vi "path steer4.vi"(11 "lane":bool) -> (2 "curve vel limit":dbl, 3 "handle":dbl=175.61695170488764)   [LabVIEW 2015]
uses:
  <vilib>/Analysis/7linalg.llb/Solve Linear Equations (single right hand).vi
  <vilib>/Analysis/baseanly.llb/Solve Linear Equations By Cholesky.vi
  <vilib>/Analysis/baseanly.llb/Real Matrix to Compact Array.vi
  <vilib>/Analysis/baseanly.llb/Real Compact Tri-Matrix Linear Eqs.vi
  G_ALL.vi
  <vilib>/Analysis/7linalg.llb/Solve Linear Eqs (General).vi
  <vilib>/Analysis/7linalg.llb/Solve Linear Eqs (Gen, single right hand).vi
  <vilib>/Analysis/NI_AALPro.lvlib
panel:
  in  "gap":dbl=3.0 format="%#_13g"
  out "cy":dbl
  out "cx":dbl
  out "slope bc":dbl
  out "slope ab":dbl
  in  "gain":dbl[](array[numeric])=[0.7, 1400.0, 750.0]
  out "R":dbl
  out "circle coeff":dbl[](array[numeric]) format="%.2f"
  out "ref":dbl[](array[numeric])
  out "circle point":dbl[][](array[numeric])
  out "map_track 2":dbl[][](array[numeric])
  in  "d lon[m] good:0.5":dbl format="%#_13g"
  out "appended array":dbl[](array[numeric])
  out "range":dbl[](graph)
  out "path end":bool
  in  "an[g]":dbl=-0.17 format="%#_13g"
  out "Waveform Graph":dynamicdata(graph)
  in  "mu":dbl=0.005 format="%#_13g"
  out "x":dbl=-0.8542483758567541
  out "XY Graph":cluster{"Y":dbl[], "Y":dbl[]}[](graph)=[{"Y"=[-5.246809304707959, -4.763210909809536, -4.298248751776158, -3.853163667485589, -3.4268765479315446, -3.029477672753705, -2.6673284986480974, -2.335336691519628, -2.0366453167866156, -1.7750835921098853, -1.5528767688369498, -1.3644656447475765, -1.2079630605299954, -1.074690008661569, -0.9585132340675446, -0.8551782329420596, -0.7665829934540727, -0.6868993462607671, -0.6126823280970868, -0.5442164343365972, -0.47614894814750475, -0.41410047141640827, -0.3538150238541624, -0.29540366128691464, -0.24219086500490516, -0.19691528446819184, -0.15547027846011519, -0.11340295527325328, -0.07144915398020535, -0.03434793001665748, 0.0, 0.026526158792223087, 0.05124494389382517, 0.07270742281515652, 0.06435385726912624, -0.004553363938687882, -0.139882839282637, -0.3359547912247316, -0.5900103181212502, -0.900040761768828, -1.2577413584671457, -1.66216965308078, -2.1012210225275174, -2.5653232377446606, -3.0450206197370466, -3.5404770109177743, -4.039369871326692, -4.541851143281866, -5.046387603513992, -5.553897537492966, -6.061637927692216, -6.567645563226444, -7.068648217182836, -7.570715384980373, -8.064438697718192, -8.545111556606587, -8.998477174205098, -9.422019565773061, -9.805695724849244, -10.146105279341642], "Y"=[-13.12635530502614, -12.964543503689939, -12.76763447744193, -12.524937360608902, -12.2475735581719, -11.933583222485607, -11.583671941038977, -11.206464906204559, -10.79245190322264, -10.354599285401152, -9.898639757724679, -9.426030687571156, -8.945680321385996, -8.454465203163156, -7.963985068856038, -7.468786738899853, -6.97312085053041, -6.479311060157665, -5.971731167568438, -5.469535412616666, -4.9636888467403155, -4.464752828537232, -3.9649913085777393, -3.458342585235778, -2.9601418499725303, -2.459972000641257, -1.9586644185731306, -1.4494467342092758, -0.9454480119816643, -0.4403687170997531, 0.06136222931732077, 0.5678735764406926, 1.068808881478275, 1.5686590067794068, 2.0720530905057277, 2.5736288544042853, 3.0594879994083963, 3.5248827445502124, 3.9579216058298154, 4.3560080630331335, 4.707794061133773, 5.011781058067703, 5.259264085768475, 5.451142759582283, 5.593309208559008, 5.693936293621469, 5.758617125078806, 5.791664966026638, 5.794000380643315, 5.784136801290129, 5.782533687658117, 5.785062966223215, 5.79993550563809, 5.8290421589798, 5.9156579447766475, 6.067163605595132, 6.278887512503447, 6.54911596168099, 6.871713294872911, 7.24413426029683]}, {"Y"=[-27.79054311036769, -27.788426793206575, -27.782078486373944, -27.77150012362555, -27.75669492723317, -27.737667407003034, -27.71442335890214, -27.686969863292695, -27.655315282775426, -27.619469259642194, -27.5794427129389, -27.5352478351394, -27.48689808843162, -27.434408200616765, -27.377794160623147, -27.317073213635787, -27.25226385584335, -27.18338582880404, -27.110460113432133, -27.033508923606977, -26.95255569940644, -26.867625099966816, -26.77874299597144, -26.68593646177021, -26.589233767132484, -26.488664368635824, -26.384258900693254, -26.2760491662217, -26.16406812695454, -26.048349893401117, -25.92892971445636, -25.805843966663623, -25.679130143134046, -25.548826842125777, -25.41497375528658, -25.27761165556337, -25.13678238478238, -24.992528840903734, -24.844894964954314, -24.693925727642892, -24.53966711566163, -24.382166117678068, -24.221470710021944, -24.057629842071115, -23.890693421341133, -23.720712298282884, -23.547738250793113, -23.37182396844231, -23.193023036425007, -23.011389919237175, -22.82697994408583, -22.639849284035826, -22.450054940898987, -22.257654727870808, -22.062707251920006, -21.865271895936253, -21.66540880064158, -21.463178846270928, -21.25864363402745, -21.05186546731817, -20.84290733277577, -20.631832881072256, -20.41870640753034, -20.20359283253847, -19.986557681775434, -19.767667066250628, -19.54698766216598, -19.324586690605734, -19.10053189706029, -18.874891530790215, -18.64773432403691, -18.419129471086073, -18.18914660719046, -17.957855787358298, -17.725327465013883, -17.491632470536747, -17.256841989686063, -17.02102754191677, -16.784260958594032, -16.546614361112756, -16.308160138928653, -16.068970927507767, -15.829119586200973, -15.588679176050324, -15.347722937533948, -15.106324268256303, -14.864556700590517, -14.622493879279771, -14.38020953900434, -14.137777481921338, -13.895271555183845, -13.652765628446353, -13.410333571363354, -13.16804923108792, -12.92598640977717, -12.684218842111388, -12.442820172833741, -12.20186393431737, -11.961423524166722, -11.721572182859921, -11.482382971439037, -11.243928749254936, -11.006282151773657, -10.769515568450924, -10.533701120681629, -10.298910639830943, -10.06521564535381, -9.832687323009392, -9.601396503177233, -9.37141363928162, -9.142808786330779, -8.915651579577474, -8.690011213307402, -8.465956419761957, -8.243555448201716, -8.022876044117066, -7.803985428592254, -7.586950277829223, -7.371836702837354, -7.158710229295436, -6.947635777591925, -6.738677643049522, -6.531899476340242, -6.32736426409676, -6.125134309726112, -5.925271214431441, -5.727835858447683, -5.53288838249688, -5.3404881694687045, -5.150693826331867, -4.96356316628186, -4.779153191130517, -4.597520073942688, -4.418719141925381, -4.242804859574576, -4.069830812084804, -3.8998496890265617, -3.7329132682965724, -3.5690724003457444, -3.4083769926896217, -3.250875994706062, -3.096617382724796, -2.9456481454133776, -2.798014269463957, -2.6537607255853093, -2.5129314548043187, -2.3755693550811117, -2.241716268241916, -2.1114129672336457, -1.9846991437040682, -1.8616133959113306, -1.7421932169665748, -1.62647498341315, -1.5144939441459915, -1.406284209674439, -1.3018787417318656, -1.201309343235204, -1.1046066485974766, -1.0118001143962498, -0.9229180104008776, -0.8379874109612526, -0.7570341867607127, -0.6800829969355568, -0.6071572815636515, -0.5382792545243404, -0.47346989673190265, -0.41274894974454135, -0.3561349097509261, -0.30364502193607024, -0.25529527522828666, -0.21110039742879394, -0.1710738507254952, -0.13522782759226182, -0.10357324707499238, -0.07611975146555316, -0.052875703364655635, -0.03384818313452165, -0.019042986742137558, -0.00846462399374559, -0.0021163171611142673, 0.0, -0.0021163171611142673, -0.00846462399374559, -0.019042986742137558, -0.03384818313452165, -0.052875703364655635, -0.07611975146555316, -0.10357324707499238, -0.13522782759226182, -0.17107385072549341, -0.21110039742879394, -0.25529527522828666, -0.30364502193607024, -0.3561349097509261, -0.4127489497445396, -0.4734698967319009, -0.5382792545243387, -0.6071572815636497, -0.6800829969355586, -0.7570341867607127, -0.8379874109612526, -0.9229180104008758, -1.011800114396248, -1.1046066485974766, -1.2013093432352022, -1.3018787417318638, -1.4062842096744355, -1.5144939441459861, -1.6264749834131482, -1.7421932169665766, -1.8616133959113323, -1.9846991437040664, -2.111412967233644, -2.2417162682419143, -2.37556935508111, -2.512931454804317, -2.6537607255853075, -2.798014269463952, -2.9456481454133705, -3.0966173827247943, -3.2508759947060604, -3.4083769926896235, -3.569072400345746, -3.7329132682965707, -3.89984968902656, -4.069830812084803, -4.242804859574575, -4.418719141925379, -4.597520073942681, -4.77915319113051, -4.9635631662818565, -5.150693826331869, -5.340488169468708, -5.532888382496882, -5.727835858447682, -5.925271214431433, -6.125134309726104, -6.3273642640967624, -6.531899476340239, -6.738677643049519, -6.947635777591917, -7.158710229295428, -7.371836702837351, -7.58695027782922, -7.803985428592251, -8.022876044117067, -8.243555448201715, -8.465956419761955, -8.6900112133074, -8.915651579577467, -9.14280878633077, -9.371413639281617, -9.601396503177229, -9.832687323009386, -10.065215645353812, -10.298910639830945, -10.533701120681625, -10.769515568450919, -11.006282151773648, -11.24392874925494, -11.482382971439037, -11.721572182859921, -11.961423524166714, -12.201863934317359, -12.442820172833729, -12.684218842111388, -12.925986409777169, -13.168049231087927, -13.410333571363354, -13.652765628446351, -13.895271555183843, -14.137777481921333, -14.380209539004332, -14.622493879279759, -14.864556700590516, -15.106324268256296, -15.347722937533955, -15.588679176050325, -15.82911958620097, -16.068970927507763, -16.30816013892865, -16.546614361112745, -16.784260958594036, -17.021027541916766, -17.25684198968606, -17.49163247053674, -17.725327465013873, -17.957855787358298, -18.189146607190455, -18.41912947108607, -18.647734324036914, -18.874891530790215, -19.100531897060286, -19.32458669060573, -19.546987662165968, -19.767667066250617, -19.986557681775434, -20.203592832538465, -20.418706407530333, -20.631832881072256, -20.842907332775766, -21.051865467318166, -21.258643634027447, -21.46317884627092, -21.66540880064158, -21.865271895936253, -22.062707251920003, -22.257654727870804, -22.45005494089898, -22.63984928403582, -22.826979944085828, -23.01138991923717, -23.19302303642501, -23.371823968442314, -23.54773825079311, -23.720712298282884, -23.890693421341126, -24.057629842071112, -24.221470710021936, -24.382166117678068, -24.539667115661626, -24.693925727642895, -24.844894964954314, -24.992528840903734, -25.13678238478238, -25.277611655563366, -25.414973755286574, -25.548826842125777, -25.679130143134046, -25.805843966663623, -25.928929714456356, -26.04834989340111, -26.16406812695454, -26.276049166221696, -26.384258900693247, -26.488664368635824, -26.589233767132484, -26.68593646177021, -26.778742995971438, -26.867625099966812, -26.95255569940643, -27.033508923606977, -27.110460113432133, -27.183385828804038, -27.25226385584335, -27.317073213635787, -27.377794160623147, -27.434408200616765, -27.486898088431616, -27.535247835139405, -27.5794427129389, -27.619469259642194, -27.655315282775426, -27.686969863292695, -27.71442335890214, -27.737667407003034, -27.75669492723317, -27.77150012362555, -27.782078486373944, -27.788426793206575], "Y"=[-0.0, -0.24250592673749302, -0.48493798382049413, -0.7272223240959237, -0.969285145406673, -1.2110527130724553, -1.4524513823501046, -1.6934076208664777, -1.9338480310171269, -2.1736993723239215, -2.4128885837448077, -2.6513428059289086, -2.8889894034101893, -3.1257559867329223, -3.3615704345022186, -3.596360915352901, -3.830055909830037, -4.062584232174453, -4.293875052006613, -4.52385791590223, -4.752462768853066, -4.97961997560637, -5.205260341876442, -5.429315135421889, -5.65171610698213, -5.872395511066782, -6.091286126591589, -6.308321277354623, -6.523434852346495, -6.736561325888409, -6.9476357775919215, -7.156593912134322, -7.363372078843605, -7.567907291087082, -7.770137245457733, -7.970000340752407, -8.167435696736161, -8.362383172686963, -8.55478338571514, -8.744577728851981, -8.931708388901985, -9.11611836405333, -9.29775148124116, -9.476552413258466, -9.652466695609267, -9.82544074309904, -9.995421866157285, -10.162358286887272, -10.326199154838099, -10.486894562494223, -10.644395560477784, -10.798654172459047, -10.949623409770469, -11.09725728571989, -11.241510829598536, -11.382340100379524, -11.519702200102733, -11.65355528694193, -11.783858587950201, -11.910572411479777, -12.033658159272512, -12.15307833821727, -12.268796571770693, -12.380777611037853, -12.488987345509406, -12.59339281345198, -12.693962211948639, -12.790664906586368, -12.883471440787595, -12.97235354478297, -13.057284144222592, -13.138237368423132, -13.215188558248288, -13.288114273620195, -13.356992300659504, -13.421801658451942, -13.482522605439303, -13.539136645432919, -13.591626533247775, -13.639976279955558, -13.684171157755053, -13.72419770445835, -13.760043727591583, -13.791698308108852, -13.819151803718292, -13.84239585181919, -13.861423372049323, -13.876228568441707, -13.8868069311901, -13.89315523802273, -13.895271555183845, -13.89315523802273, -13.8868069311901, -13.876228568441707, -13.861423372049323, -13.84239585181919, -13.819151803718293, -13.791698308108852, -13.760043727591583, -13.72419770445835, -13.684171157755053, -13.639976279955558, -13.591626533247775, -13.53913664543292, -13.482522605439303, -13.421801658451942, -13.356992300659504, -13.288114273620195, -13.215188558248288, -13.138237368423134, -13.057284144222592, -12.972353544782969, -12.883471440787595, -12.790664906586368, -12.69396221194864, -12.593392813451981, -12.488987345509406, -12.380777611037855, -12.268796571770697, -12.153078338217272, -12.033658159272516, -11.910572411479778, -11.783858587950201, -11.65355528694193, -11.519702200102735, -11.382340100379528, -11.241510829598536, -11.09725728571989, -10.949623409770469, -10.79865417245905, -10.644395560477784, -10.486894562494225, -10.326199154838102, -10.162358286887274, -9.995421866157285, -9.825440743099042, -9.65246669560927, -9.476552413258466, -9.297751481241159, -9.11611836405333, -8.931708388901988, -8.74457772885198, -8.554783385715142, -8.362383172686968, -8.167435696736163, -7.9700003407524065, -7.770137245457734, -7.567907291087087, -7.363372078843605, -7.1565939121343245, -6.9476357775919215, -6.7365613258884105, -6.523434852346494, -6.308321277354625, -6.091286126591593, -5.872395511066783, -5.6517161069821285, -5.42931513542189, -5.205260341876445, -4.979619975606376, -4.752462768853069, -4.523857915902228, -4.293875052006615, -4.062584232174458, -3.8300559098300377, -3.596360915352905, -3.361570434502219, -3.1257559867329254, -2.888989403410189, -2.6513428059289113, -2.4128885837448126, -2.1736993723239233, -1.933848031017125, -1.6934076208664786, -1.4524513823501084, -1.2110527130724555, -0.969285145406676, -0.7272223240959296, -0.4849379838204965, -0.24250592673749197, -1.7016237834565482e-15, 0.24250592673748858, 0.4849379838204931, 0.72722232409592, 0.9692851454066664, 1.2110527130724522, 1.4524513823501048, 1.6934076208664814, 1.9338480310171278, 2.1736993723239197, 2.4128885837448095, 2.6513428059289077, 2.8889894034101857, 3.1257559867329223, 3.3615704345022155, 3.5963609153528955, 3.830055909830029, 4.062584232174455, 4.293875052006618, 4.523857915902231, 4.752462768853065, 4.979619975606372, 5.205260341876442, 5.429315135421887, 5.651716106982125, 5.872395511066779, 6.0912861265915845, 6.308321277354616, 6.52343485234649, 6.736561325888413, 6.947635777591924, 7.156593912134322, 7.363372078843602, 7.567907291087084, 7.7701372454577315, 7.970000340752404, 8.16743569673616, 8.36238317268696, 8.554783385715135, 8.744577728851977, 8.931708388901985, 9.116118364053332, 9.29775148124116, 9.476552413258464, 9.652466695609267, 9.825440743099039, 9.995421866157281, 10.162358286887272, 10.326199154838095, 10.48689456249422, 10.644395560477783, 10.798654172459052, 10.94962340977047, 11.09725728571989, 11.241510829598534, 11.382340100379523, 11.51970220010273, 11.653555286941932, 11.7838585879502, 11.910572411479777, 12.03365815927251, 12.153078338217266, 12.268796571770695, 12.380777611037853, 12.488987345509404, 12.593392813451981, 12.69396221194864, 12.790664906586366, 12.883471440787595, 12.972353544782967, 13.057284144222589, 13.138237368423132, 13.215188558248288, 13.288114273620193, 13.356992300659506, 13.421801658451942, 13.482522605439303, 13.539136645432919, 13.591626533247773, 13.63997627995556, 13.684171157755053, 13.72419770445835, 13.760043727591581, 13.791698308108852, 13.819151803718292, 13.84239585181919, 13.861423372049323, 13.876228568441707, 13.8868069311901, 13.89315523802273, 13.895271555183845, 13.89315523802273, 13.8868069311901, 13.876228568441707, 13.861423372049323, 13.84239585181919, 13.819151803718292, 13.791698308108852, 13.760043727591583, 13.724197704458351, 13.684171157755053, 13.63997627995556, 13.591626533247773, 13.539136645432919, 13.482522605439305, 13.421801658451944, 13.356992300659506, 13.288114273620195, 13.21518855824829, 13.138237368423134, 13.05728414422259, 12.972353544782969, 12.883471440787597, 12.79066490658637, 12.693962211948643, 12.593392813451985, 12.488987345509408, 12.380777611037855, 12.268796571770697, 12.15307833821727, 12.033658159272512, 11.910572411479778, 11.783858587950203, 11.653555286941934, 11.519702200102733, 11.382340100379524, 11.241510829598537, 11.097257285719893, 10.949623409770474, 10.798654172459056, 10.644395560477784, 10.486894562494227, 10.326199154838095, 10.16235828688727, 9.995421866157285, 9.825440743099042, 9.65246669560927, 9.47655241325847, 9.29775148124117, 9.11611836405333, 8.931708388901988, 8.744577728851976, 8.554783385715139, 8.362383172686963, 8.167435696736165, 7.970000340752413, 7.770137245457741, 7.567907291087083, 7.363372078843606, 7.156593912134326, 6.947635777591929, 6.736561325888418, 6.523434852346495, 6.308321277354626, 6.091286126591594, 5.872395511066778, 5.65171610698213, 5.429315135421891, 5.205260341876446, 4.979619975606377, 4.752462768853076, 4.52385791590223, 4.293875052006616, 4.062584232174459, 3.8300559098300337, 3.5963609153529004, 3.3615704345022204, 3.125755986732927, 2.888989403410197, 2.651342805928907, 2.4128885837448086, 2.173699372323925, 1.9338480310171329, 1.6934076208664863, 1.4524513823501162, 1.2110527130724573, 0.9692851454066778, 0.7272223240959189, 0.484937983820492, 0.24250592673749366]}]
  # "d lon : 경로 위 3점 위치 밀기"
  # "mu : 마찰력\nan :  감가속도"
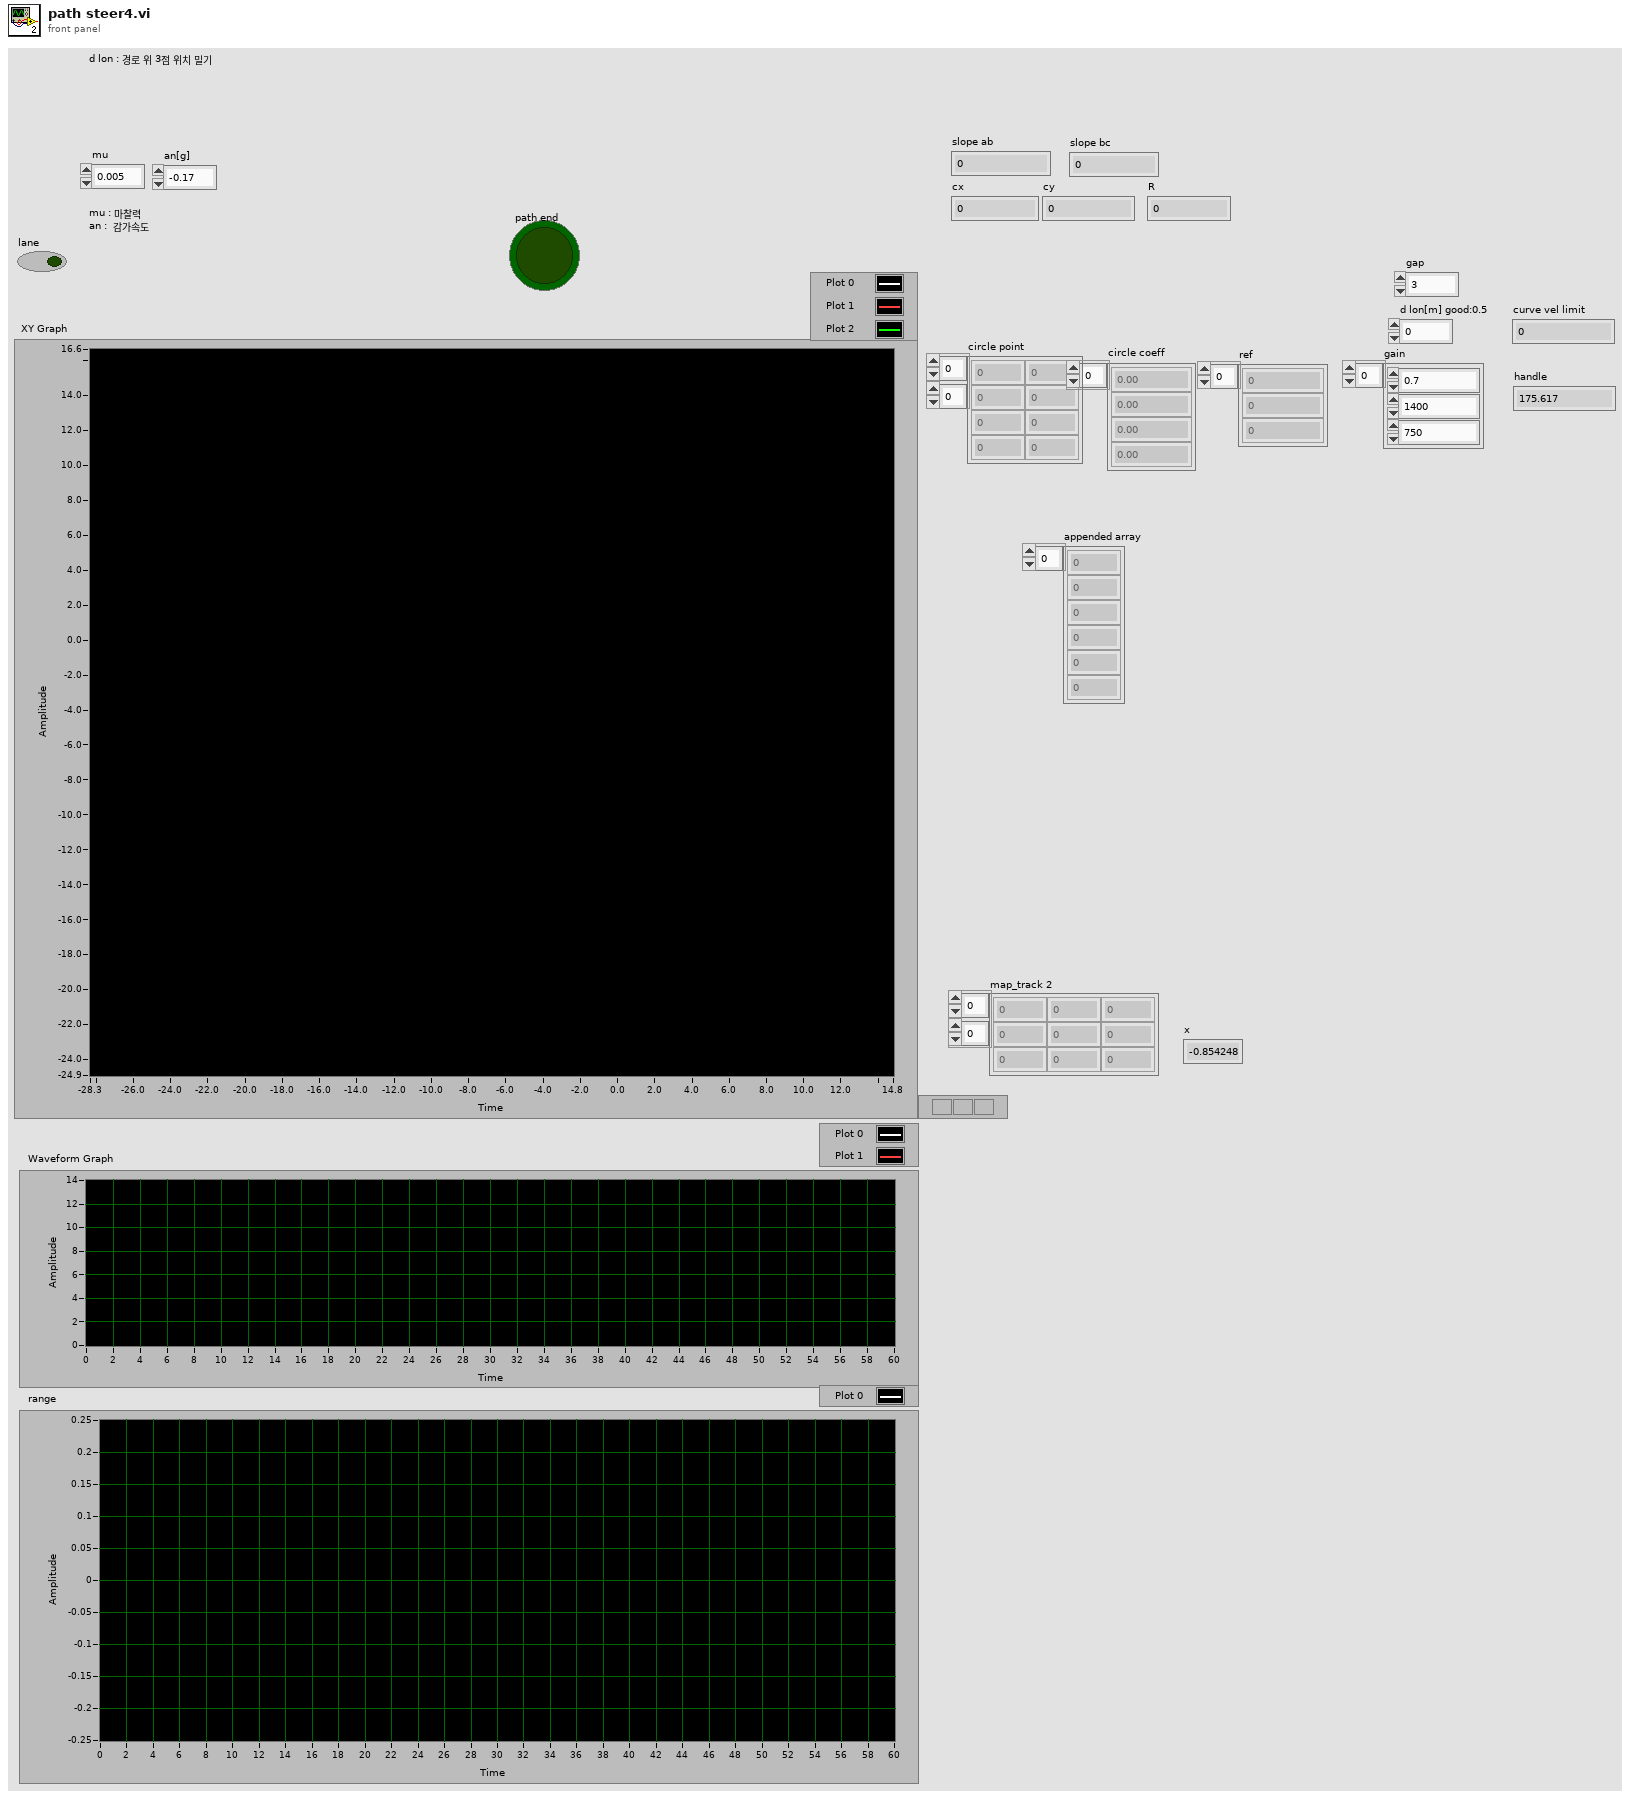
[diagram p1: front panel]
types:
  T1 = cluster{"Steer_input":dbl, "Steer_output":dbl, "VS_des":dbl, "VS_can":dbl, "heading":dbl, "auto":bool, "run":bool, "x":dbl, "y":dbl, "slam_y":dbl, "slam_x":dbl, "slam_heading":dbl}
  T2 = cluster{"C_Wheel base":dbl, "ratio_steer":dbl, "Overall width":dbl, "af":dbl, "turn radius":dbl, "eval":dbl, "ap":dbl, "an":dbl, "Vmax":dbl, "mu":dbl, "Vlast":dbl}
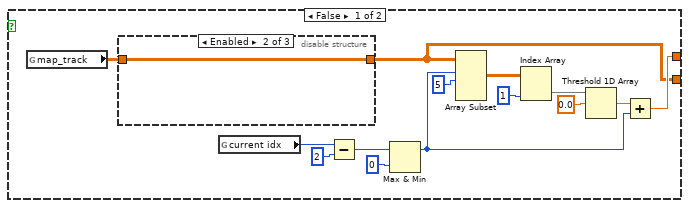
[diagram p2: hidden frame]
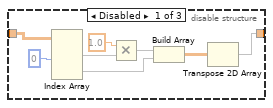
[diagram p3: hidden frame]
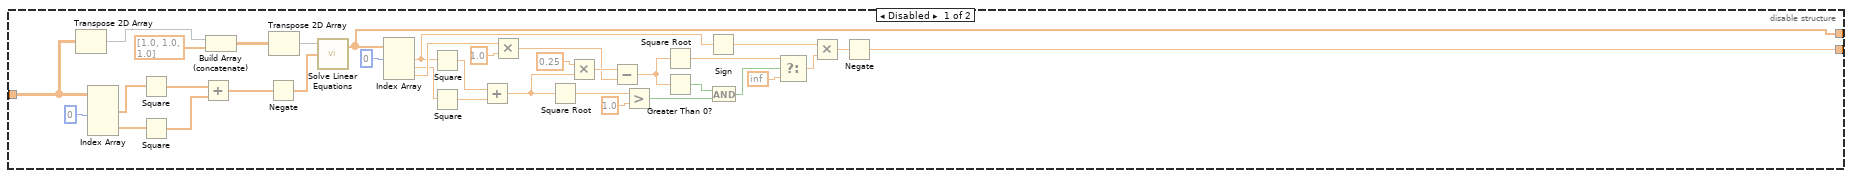
[diagram p6: hidden frame]
diagram:
  n1 = flat-sequence {
    tunnel: [w10] -> w9
    tunnel: w9 -> [w111]
    tunnel: [w124] -> w8
    tunnel: [w118] -> w7
    tunnel: [w111] -> w6
    tunnel: w8 -> [w279]
    tunnel: [w279] -> w5
    tunnel: w7 -> [w278]
    tunnel: [w278] -> w3
    tunnel: w6 -> [w264]
    tunnel: w5 -> [w458]
    tunnel: [w458] -> w4
    tunnel: w3 -> [w457]
    tunnel: [w457] -> w2
    tunnel: [w418] -> w1
    tunnel: w4 -> [w461]
    tunnel: w2 -> [w460]
    tunnel: w1 -> [w459]
    frame #0 {
      n2 = case shown="True" "lane" {
        tunnel: [w66 w89] -> w56
        tunnel: [w68 _] -> w19
        frame False {
          n3 = global read "G_ALL.vi" "map_track"() -> (w67:dbl[][])
          n4 = disable-structure shown="Enabled" {
            disable-tunnel: w67 -> [w87 w88 _]
            disable-tunnel: [w80 w88 _] -> w66
            frame Disabled {
              n5 = Index Array(array=w87, index (col) #1=0 ("disabled index (col)")) -> (element #1=w85:dbl[], element #2=w82:dbl[])  [unwired: 3 in]
              n6 = Multiply(x=1.0, y=w85) -> (x*y=w83:dbl[])
              n7 = Build Array(w83, w82) -> (w81:dbl[][])
              n8 = Transpose 2D Array(2D array=w81) -> (transposed array=w80:dbl[][])
            }
            frame Enabled {
            }
            frame Disabled {
            }
          }
          n9 = global read "G_ALL.vi" "current idx"() -> (w69:i32)
          n10 = Subtract(x=w69, y=2) -> (x-y=w78:i32)
          n11 = Max & Min(x=w78, y=0) -> (max(x,y)=w72:i32)  [unwired: 1 out]
          n12 = Array Subset(array=w66, index (row)=w72, length (row)=5 ("length")) -> (w75:dbl[][])  [unwired: 2 in]
          n13 = Index Array(array=w75, index (col)=1 ("disabled index (col)")) -> (element=w73:dbl[])  [unwired: 1 in]
          n14 = Threshold 1D Array(2:0.0 ("threshold y"), 3:w73) -> (0:w70:dbl)  [unwired: 1 in]
          n15 = Add(x=w70, y=w72) -> (x+y=w68:dbl)
        }
        frame True {
          n16 = global read "G_ALL.vi" "map_track lane"() -> (w89:dbl[][])
        }
      }
      n17 = Round Toward +Infinity(x=w19) -> (ceil(x): smallest int >= x=w27:dbl)
      n18 = Round Toward -Infinity(1:w19) -> (0:w26:dbl)
      n19 = Index Array(array=w56, index (col) #1=0 ("disabled index (col)")) -> (element #1=w64:dbl[], element #2=w63:dbl[])  [unwired: 3 in]
      n20 = Equal?(x=w26, y=w19) -> (x = y?=w25:bool)
      n21 = To Long Integer(number=w26) -> (32bit integer=w23:i32)
      n22 = Interpolate 1D Array(1:w19, 2:w64) -> (0:w62:dbl)
      n23 = Interpolate 1D Array(1:w19, 2:w63) -> (0:w61:dbl)
      n24 = Increment(x=w23) -> (x+1=w22:i32)
      n25 = To Long Integer(number=w27) -> (32bit integer=w21:i32)
      n26 = Select(t=w23, s=w25, f=w22) -> (s? t:f=w24:i32)
      n27 = global read "G_ALL.vi" "CARDATA"() -> (w58:T1)
      n28 = Array Subset(array=w56, index (row)=0 ("index"), length (row)=w24) -> (w54:dbl[][])  [unwired: 2 in]
      n29 = Unbundle By Name(w58) -> ("VS_can"=w18:dbl)
      n30 = Index Array(array=w54, index (col) #1=0 ("disabled index (col)")) -> (element #1=w52:dbl[], element #2=w51:dbl[])  [unwired: 3 in]
      n31 = Reverse 1D Array(array=w52) -> (reversed array=w50:dbl[])
      n32 = Reverse 1D Array(array=w51) -> (reversed array=w49:dbl[])
      n33 = Multiply(x=2.0, y=w18) -> (x*y=w17:dbl)
      n34 = Build Array(w50, w49) -> (w29:dbl[][])
      n35 = Max & Min(x=w17, y=25.0) -> (max(x,y)=w57:dbl)  [unwired: 1 out]
      n36 = Transpose 2D Array(2D array=w29) -> (transposed array=w28:dbl[][])
      n37 = Build Array(w62, w61) -> (w47:dbl[])
      n38 = Array Subset(array=w56, index (row)=w21) -> (w31:dbl[][])  [unwired: 3 in]
      n39 = for {
        tunnel: w28 -> [w92] mode=indexing
        shift-right: [w92] -> _
        shift-left: w47 -> [w99]
        shift-right: [w91] -> _
        shift-left: 0.0 -> [w94]
        tunnel: 15.0 ("y") -> [w93]
        tunnel: [w91] -> w43 mode=indexing
        stop <- w90 stop-if-true
        n40 = Subtract(x=w92, y=w99) -> (x-y=w98:dbl[])
        n41 = Square(x=w98) -> (x^2=w97:dbl[])
        n42 = Add Array Elements(numeric array=w97) -> (sum=w96:dbl)
        n43 = Square Root(x=w96) -> (sqrt(x)=w95:dbl)
        n44 = Add(x=w94, y=w95) -> (x+y=w91:dbl)
        n45 = Greater Or Equal?(x=w91, y=w93) -> (x >= y?=w90:bool)
      }
      n46 = for {
        tunnel: w31 -> [w102] mode=indexing
        shift-right: [w102] -> _
        shift-left: w47 -> [w109]
        shift-right: [w101] -> _
        shift-left: 0.0 -> [w104]
        tunnel: w57 -> [w103]
        tunnel: [w101] -> w30 mode=indexing
        tunnel: [w100] -> w13
        stop <- w100 stop-if-true
        n47 = Subtract(x=w102, y=w109) -> (x-y=w108:dbl[])
        n48 = Square(x=w108) -> (x^2=w107:dbl[])
        n49 = Add Array Elements(numeric array=w107) -> (sum=w106:dbl)
        n50 = Square Root(x=w106) -> (sqrt(x)=w105:dbl)
        n51 = Add(x=w104, y=w105) -> (x+y=w101:dbl)
        n52 = Greater Or Equal?(x=w101, y=w103) -> (x >= y?=w100:bool)
      }
      n53 = Not(x=w13) -> (.not. x?=→"path end":bool)
      n54 = Negate(x=w43) -> (-x=w45:dbl[])
      n55 = Array Size(array=w43) -> (size(s)=w41:i32)
      n56 = Array Size(array=w30) -> (size(s)=w14:i32)
      n57 = Reverse 1D Array(array=w45) -> (reversed array=w44:dbl[])
      n58 = Array Subset(array=w28, index (row)=0 ("index"), length (row)=w41) -> (w36:dbl[][])  [unwired: 2 in]
      n59 = Array Subset(array=w31, index (row)=0 ("index"), length (row)=w14) -> (w15:dbl[][])  [unwired: 2 in]
      n60 = Build Array (concatenate)(w44, w30) -> (w10:dbl[])
      n61 = Index Array(array=w36, index (col) #1=0 ("disabled index (col)")) -> (element #1=w35:dbl[], element #2=w34:dbl[])  [unwired: 3 in]
      n62 = Reverse 1D Array(array=w35) -> (reversed array=w38:dbl[])
      n63 = Reverse 1D Array(array=w34) -> (reversed array=w39:dbl[])
      n64 = Build Array(w38, w39) -> (w40:dbl[][])
      n65 = Transpose 2D Array(2D array=w40) -> (transposed array=w33:dbl[][])
      n66 = Build Array (concatenate)(w33, w15) -> (w11:dbl[][])
      "map_track 2" <- w11
      n67 = global write "G_ALL.vi" "dist"(w10) -> ()
      n68 = global write "G_ALL.vi" "map_track 2"(w11) -> ()
    }
    frame #1 {
      n69 = Threshold 1D Array(2:0.0 ("threshold y"), 3:w111) -> (0:w152:dbl)  [unwired: 1 in]
      n70 = local read "map_track 2"() -> (w110:dbl[][])
      n71 = Index Array(array=w110, index (col) #1=0 ("disabled index (col)"), index (col) #3=0 ("index (col)")) -> (element #1=w159:dbl[], element #2=w151:dbl[], element #3=w149:dbl[])  [unwired: 4 in]
      n72 = Array Size(array=w151) -> (size(s)=w158:i32)
      n73 = Interpolate 1D Array(1:w152, 2:w149) -> (0:→"x":dbl)
      n74 = Decrement(x=w158) -> (x-1=w157:i32)
      n75 = for {
        tunnel: w111 -> [w194]
        tunnel: w111 -> [w239] mode=indexing
        tunnel: w159 -> [w191]
        tunnel: w151 -> [w190]
        tunnel: [w207] -> w156 mode=indexing
        tunnel: w157 -> [w206]
        tunnel: [w184] -> w155 mode=indexing
        tunnel: [w187] -> w115
        tunnel: 5.0 ("x") -> [w192]
        tunnel: [w186] -> _ mode=indexing
        i -> [w187]
        stop <- w205 stop-if-true
        n76 = Add(x=w239, y=w192) -> (x+y=w186:dbl)
        n77 = Add(x=w186, y=w192) -> (x+y=w193:dbl)
        n78 = Index Array(array=w191, index=w187) -> (element=w233:dbl)
        n79 = Index Array(array=w190, index=w187) -> (element=w232:dbl)
        n80 = Threshold 1D Array(1:w187, 2:w186, 3:w194) -> (0:w238:dbl)
        n81 = Threshold 1D Array(1:w187, 2:w193, 3:w194) -> (0:w188:dbl)
        n82 = Interpolate 1D Array(1:w238, 2:w191) -> (0:w185:dbl)
        n83 = Interpolate 1D Array(1:w238, 2:w190) -> (0:w237:dbl)
        n84 = Greater Or Equal?(x=w188, y=w206) -> (x >= y?=w205:bool)
        n85 = Interpolate 1D Array(1:w188, 2:w191) -> (0:w236:dbl)
        n86 = Interpolate 1D Array(1:w188, 2:w190) -> (0:w235:dbl)
        n87 = Build Array(w233, w232) -> (w201:dbl[])
        n88 = Build Array(w236, w235) -> (w234:dbl[])
        n89 = Build Array(w185, w237) -> (w189:dbl[])
        n90 = Build Array(w201, w189, w234) -> (w204:dbl[][])
        n91 = Build Array(w189, w189, w189) -> (w203:dbl[][])
        n92 = Subtract(x=w204, y=w203) -> (x-y=w202:dbl[][])
        n93 = Transpose 2D Array(2D array=w202) -> (transposed array=w213:dbl[][])
        n94 = Index Array(array=w202, index (col) #1=0 ("disabled index (col)")) -> (element #1=w209:dbl[], element #2=w210:dbl[])  [unwired: 3 in]
        n95 = Square(x=w209) -> (x^2=w211:dbl[])
        n96 = Square(x=w210) -> (x^2=w212:dbl[])
        n97 = Add(x=w211, y=w212) -> (x+y=w214:dbl[])
        n98 = Build Array (concatenate)(w213, dbl[] [1.0, 1.0, 1.0] ("initialized array")) -> (w223:dbl[][])
        n99 = Negate(x=w214) -> (-x=w215:dbl[])
        n100 = Transpose 2D Array(2D array=w223) -> (transposed array=w224:dbl[][])
        n101 = call-poly <vilib>:"Solve Linear Equations.vi"("Known Vector"=w215, "Input Matrix"=w224) -> ("Solution Vector"=w216:dbl[])  [unwired: 1 in, 1 out]
        n102 = Index Array(array=w216, index #1=0 ("index")) -> (element #1=w184:dbl, element #2=w218:dbl, element #3=w221:dbl)  [unwired: 2 in]
        n103 = Square(x=w184) -> (x^2=w219:dbl)
        n104 = Square(x=w218) -> (x^2=w220:dbl)
        n105 = Add(x=w219, y=w220) -> (x+y=w200:dbl)
        n106 = Multiply(x=w221, y=1.0) -> (x*y=w222:dbl)
        n107 = Square Root(x=w200) -> (sqrt(x)=w199:dbl)
        n108 = Multiply(x=0.25, y=w200) -> (x*y=w229:dbl)
        n109 = Subtract(x=w229, y=w222) -> (x-y=w225:dbl)
        n110 = Greater?(x=w199, y=1.0) -> (0:w196:bool)
        n111 = Greater Than 0?(x=w225) -> (x > 0?=w197:bool)
        n112 = Square Root(x=w225) -> (sqrt(x)=w231:dbl)
        n113 = And(x=w197, y=w196) -> (x .and. y?=w195:bool)
        n114 = Select(t=w231, s=w195, f=inf) -> (s? t:f=w207:dbl)
      }
      n115 = Threshold 1D Array(2:0.0 ("threshold y"), 3:w111) -> (0:w112:dbl)  [unwired: 1 in]
      n116 = Array Subset(array=w155, length=w115) -> (w154:dbl[])  [unwired: 1 in]
      n117 = Array Subset(array=w156, length=w115) -> (w138:dbl[])  [unwired: 1 in]
      n118 = Array Subset(array=w111, length=w115) -> (w131:dbl[])  [unwired: 1 in]
      n119 = local read "mu"() -> (w139:dbl)
      n120 = Sign(1:w154) -> (0:w116:dbl[])
      n121 = Multiply(x=w116, y=w138) -> (x*y=w137:dbl[])
      n122 = Compound Arithmetic op=MULTIPLY(w138, 9.81 ("value"), w139) -> (w141:dbl[])
      n123 = Reciprocal(x=w137) -> (1/x=w113:dbl[])
      "range" <- w113
      n124 = Square Root(x=w141) -> (sqrt(x)=w119:dbl[])
      n125 = Max & Min(x=w119, y=56.0 ("value")) -> (min(x,y)=w118:dbl[])  [unwired: 1 out]
      n126 = Interpolate 1D Array(1:w112, 2:w113) -> (0:w114:dbl)
      n127 = local read "path end"() -> (w128:bool)
      n128 = Reciprocal(x=w114) -> (1/x=w120:dbl)
      n129 = Reverse 1D Array(array=w118) -> (reversed array=w127:dbl[])
      n130 = Absolute Value(x=w120) -> (abs(x)=w142:dbl)
      n131 = case shown="True" w128 {
        tunnel: w127 -> [w161 w165]
        tunnel: [w161 w164] -> w126
        frame False {
        }
        frame True {
          n132 = Replace Array Subset(array=w165, new element=0.0 ("new element/subarray"), index=0) -> (w164:dbl[])
        }
      }
      n133 = Reverse 1D Array(array=w131) -> (reversed array=w136:dbl[])
      n134 = Compound Arithmetic op=MULTIPLY(w142, 9.81 ("value"), "mu") -> (w145:dbl)
      n135 = Array Size(array=w126) -> (size(s)=w132:i32)
      n136 = Decrement(x=w132) -> (x-1=w134:i32)
      n137 = Negate(x=w136) -> (-x=w135:dbl[])
      n138 = Square Root(x=w145) -> (sqrt(x)=w123:dbl)
      n139 = for {
        N: w134 -> [_]
        tunnel: w126 -> [w181] mode=indexing
        tunnel: w135 -> [w182]
        shift-right: [w172] -> w133
        shift-left: w126 -> [w175]
        tunnel: w135 -> [w169] mode=indexing
        tunnel: "an[g]" -> [w166]
        i -> [w183]
        n140 = Square(x=w181) -> (x^2=w180:dbl)
        n141 = Increment(x=w183) -> (x+1=w174:i32)
        n142 = Array Subset(array=w175, index=w174) -> (w176:dbl[])  [unwired: 1 in]
        n143 = Array Subset(array=w182, index=w174) -> (w170:dbl[])  [unwired: 1 in]
        n144 = Subtract(x=w170, y=w169) -> (x-y=w168:dbl[])
        n145 = Compound Arithmetic op=MULTIPLY(w168, 9.81 ("value"), 2.0 ("value"), w166) -> (w178:dbl[])
        n146 = Subtract(x=w180, y=w178) -> (x-y=w177:dbl[])
        n147 = Square Root(x=w177) -> (sqrt(x)=w171:dbl[])
        n148 = Max & Min(x=w176, y=w171) -> (min(x,y)=w173:dbl[])  [unwired: 1 out]
        n149 = Replace Array Subset(array=w175, new element=w173, index=w174) -> (w172:dbl[])
      }
      n150 = Reverse 1D Array(array=w133) -> (reversed array=w124:dbl[])
      n151 = Interpolate 1D Array(1:w112, 2:w124) -> (0:w122:dbl)
      n152 = Max & Min(x=w123, y=w122) -> (min(x,y)=w129:dbl)  [unwired: 1 out]
      n153 = Multiply(x=w129, y=3.6) -> (x*y=→"curve vel limit":dbl)
    }
    frame #2 {
      n154 = local read "range"() -> (w263:dbl[])
      n155 = Negate(x="gap") -> (-x=w243:dbl)
      n156 = global read "G_ALL.vi" "map_track 2"() -> (w272:dbl[][])
      n157 = Subtract(x="d lon[m] good:0.5", y=0.25) -> (x-y=w240:dbl)
      n158 = In Range and Coerce(upper limit=0.01, x=w263, lower limit=-0.01) -> (In Range?=w265:bool[])  [unwired: 1 out]
      n159 = Add(x=w240, y="gap") -> (x+y=w256:dbl)
      n160 = Add(x=w243, y=w240) -> (x+y=w257:dbl)
      n161 = Add(x=0.0 ("f"), y=w240) -> (x+y=w254:dbl)
      n162 = Threshold 1D Array(2:w256, 3:w264) -> (0:w261:dbl)  [unwired: 1 in]
      n163 = Threshold 1D Array(2:w254, 3:w264) -> (0:w262:dbl)  [unwired: 1 in]
      n164 = Threshold 1D Array(2:w257, 3:w264) -> (0:w259:dbl)  [unwired: 1 in]
      n165 = Boolean To (0,1)(Boolean=w265) -> (0, 1=w260:i16[])
      n166 = Index Array(array=w272, index (col) #1=0 ("disabled index (col)")) -> (element #1=w267:dbl[], element #2=w266:dbl[])  [unwired: 3 in]
      n167 = Interpolate 1D Array(1:w261, 2:w260) -> (0:w251:dbl)
      n168 = Interpolate 1D Array(1:w262, 2:w260) -> (0:w252:dbl)
      n169 = Interpolate 1D Array(1:w259, 2:w260) -> (0:w253:dbl)
      n170 = Interpolate 1D Array(1:w261, 2:w267) -> (0:w268:dbl)
      n171 = Interpolate 1D Array(1:w261, 2:w266) -> (0:w269:dbl)
      n172 = Interpolate 1D Array(1:w262, 2:w267) -> (0:w274:dbl)
      n173 = Interpolate 1D Array(1:w262, 2:w266) -> (0:w273:dbl)
      n174 = Interpolate 1D Array(1:w259, 2:w267) -> (0:w271:dbl)
      n175 = Interpolate 1D Array(1:w259, 2:w266) -> (0:w270:dbl)
      n176 = Build Array(w251, w252, w253) -> (→"appended array":dbl[])
      n177 = Build Array(w268, w269) -> (w248:dbl[])
      n178 = Build Array(w274, w273) -> (w250:dbl[])
      n179 = Build Array(w271, w270) -> (w249:dbl[])
      n180 = Build Array(w248, w250, w249) -> (w247:dbl[][])
      "circle point" <- w247
      n181 = disable-structure shown="Enabled" {
        disable-tunnel: w247 -> [w282 w321]
        disable-tunnel: [w281 w316] -> w246
        disable-tunnel: [w280 w317] -> w245
        frame Disabled {
          n182 = Transpose 2D Array(2D array=w282) -> (transposed array=w299:dbl[][])
          n183 = Index Array(array=w282, index (col) #1=0 ("disabled index (col)")) -> (element #1=w295:dbl[], element #2=w296:dbl[])  [unwired: 3 in]
          n184 = Square(x=w295) -> (x^2=w297:dbl[])
          n185 = Square(x=w296) -> (x^2=w298:dbl[])
          n186 = Add(x=w297, y=w298) -> (x+y=w300:dbl[])
          n187 = Build Array (concatenate)(w299, dbl[] [1.0, 1.0, 1.0] ("initialized array")) -> (w307:dbl[][])
          n188 = Negate(x=w300) -> (-x=w301:dbl[])
          n189 = Transpose 2D Array(2D array=w307) -> (transposed array=w308:dbl[][])
          n190 = call-poly <vilib>:"Solve Linear Equations.vi"("Known Vector"=w301, "Input Matrix"=w308) -> ("Solution Vector"=w281:dbl[])  [unwired: 1 in, 1 out]
          n191 = Index Array(array=w281, index #1=0 ("index")) -> (element #1=w284:dbl, element #2=w283:dbl, element #3=w305:dbl)  [unwired: 2 in]
          n192 = Square(x=w284) -> (x^2=w303:dbl)
          n193 = Square(x=w283) -> (x^2=w304:dbl)
          n194 = Add(x=w303, y=w304) -> (x+y=w293:dbl)
          n195 = Multiply(x=w305, y=1.0) -> (x*y=w306:dbl)
          n196 = Square Root(x=w293) -> (sqrt(x)=w292:dbl)
          n197 = Multiply(x=0.25, y=w293) -> (x*y=w313:dbl)
          n198 = Subtract(x=w313, y=w306) -> (x-y=w309:dbl)
          n199 = Greater?(x=w292, y=1.0) -> (0:w289:bool)
          n200 = Square Root(x=w309) -> (sqrt(x)=w315:dbl)
          n201 = Greater Than 0?(x=w309) -> (x > 0?=w290:bool)
          n202 = Sign(1:w284) -> (0:w287:dbl)
          n203 = And(x=w290, y=w289) -> (x .and. y?=w288:bool)
          n204 = Select(t=w315, s=w288, f=inf) -> (s? t:f=w285:dbl)
          n205 = Multiply(x=w287, y=w285) -> (x*y=w286:dbl)
          n206 = Negate(x=w286) -> (-x=w280:dbl)
        }
        frame Enabled {
          n207 = flat-sequence {
            tunnel: w321 -> [w322]
            tunnel: [w322] -> w320
            tunnel: w320 -> [w341]
            tunnel: [w341] -> w319
            tunnel: w319 -> [w373]
            tunnel: [w373] -> w318
            tunnel: w318 -> [w414]
            tunnel: [w394] -> w317
            tunnel: [w395] -> w316
            frame #0 {
              n208 = Index Array(array=w322, index (col) #1=1 ("disabled index (col)"), index (col) #2=0 ("index (col)")) -> (element #1=w338:dbl[], element #2=w329:dbl[])  [unwired: 2 in]
              n209 = Index Array(array=w338, index #1=0 ("index")) -> (element #1=w336:dbl, element #2=w335:dbl, element #3=w334:dbl)  [unwired: 2 in]
              n210 = Index Array(array=w329, index #1=0 ("index")) -> (element #1=w331:dbl, element #2=w332:dbl, element #3=w333:dbl)  [unwired: 2 in]
              n211 = Subtract(x=w336, y=w335) -> (x-y=w328:dbl)
              n212 = Subtract(x=w335, y=w334) -> (x-y=w326:dbl)
              n213 = Subtract(x=w331, y=w332) -> (x-y=w327:dbl)
              n214 = Subtract(x=w332, y=w333) -> (x-y=w325:dbl)
              n215 = Divide(x=w328, y=w327) -> (x/y=→"slope ab":dbl)
              n216 = Divide(x=w326, y=w325) -> (x/y=→"slope bc":dbl)
            }
            frame #1 {
              n217 = Index Array(array=w341, index (col) #1=0 ("disabled index (col)"), index (col) #2=1 ("index (col)")) -> (element #1=w371:dbl[], element #2=w358:dbl[])  [unwired: 2 in]
              n218 = Index Array(array=w358, index #1=2 ("index"), index #2=0 ("index")) -> (element #1=w355:dbl, element #2=w354:dbl)
              n219 = Index Array(array=w371, index #1=2 ("index"), index #2=1 ("index"), index #3=0 ("index")) -> (element #1=w366:dbl, element #2=w363:dbl, element #3=w362:dbl)
              n220 = Subtract(x=w355, y=w354) -> (x-y=w345:dbl)
              n221 = local read "slope ab"() -> (w365:dbl)
              n222 = local read "slope bc"() -> (w344:dbl)
              n223 = local read "slope ab"() -> (w343:dbl)
              n224 = local read "slope bc"() -> (w352:dbl)
              n225 = Add(x=w366, y=w363) -> (x+y=w364:dbl)
              n226 = Add(x=w363, y=w362) -> (x+y=w361:dbl)
              n227 = Multiply(x=w365, y=w364) -> (x*y=w360:dbl)
              n228 = Multiply(x=w361, y=w344) -> (x*y=w359:dbl)
              n229 = Subtract(x=w343, y=w352) -> (x-y=w351:dbl)
              n230 = Compound Arithmetic op=MULTIPLY(w344, w345, w343) -> (w342:dbl)
              n231 = Subtract(x=w360, y=w359) -> (x-y=w353:dbl)
              n232 = Multiply(x=w351, y=2.0) -> (x*y=w348:dbl)
              n233 = Add(x=w353, y=w342) -> (x+y=w349:dbl)
              n234 = Divide(x=w349, y=w348) -> (x/y=→"cx":dbl)
            }
            frame #2 {
              n235 = Index Array(array=w373, index (col) #1=0 ("index (row)")) -> (element #1=w392:dbl[], element #2=w377:dbl[])  [unwired: 3 in]
              n236 = Index Array(array=w392, index #1=0 ("index")) -> (element #1=w390:dbl, element #2=w389:dbl)  [unwired: 1 in]
              n237 = Index Array(array=w377, index #1=0 ("index")) -> (element #1=w379:dbl, element #2=w380:dbl)  [unwired: 1 in]
              n238 = Add(x=w390, y=w389) -> (x+y=w388:dbl)
              n239 = Add(x=w379, y=w380) -> (x+y=w381:dbl)
              n240 = local read "slope ab"() -> (w393:dbl)
              n241 = Multiply(x=w388, y=0.5) -> (x*y=w386:dbl)
              n242 = local read "cx"() -> (w385:dbl)
              n243 = Reciprocal(x=w393) -> (1/x=w383:dbl)
              n244 = Subtract(x=w386, y=w385) -> (x-y=w384:dbl)
              n245 = Multiply(x=w383, y=w384) -> (x*y=w376:dbl)
              n246 = Multiply(x=w381, y=0.5) -> (x*y=w375:dbl)
              n247 = Add(x=w376, y=w375) -> (x+y=→"cy":dbl)
            }
            frame #3 {
              n248 = local read "cx"() -> (w408:dbl)
              n249 = Index Array(array=w414, index (row)=0) -> (element=w409:dbl[])  [unwired: 1 in]
              n250 = Sign(1:w408) -> (0:w407:dbl)
              n251 = local read "cy"() -> (w412:dbl)
              n252 = Build Array(w408, w412) -> (w405:dbl[])
              n253 = Subtract(x=w405, y=w409) -> (x-y=w411:dbl[])
              n254 = local read "cx"() -> (w403:dbl)
              n255 = local read "cy"() -> (w402:dbl)
              n256 = Square(x=w411) -> (x^2=w410:dbl[])
              n257 = Square(x=w403) -> (x^2=w401:dbl)
              n258 = Square(x=w402) -> (x^2=w400:dbl)
              n259 = Add(x=w401, y=w400) -> (x+y=w399:dbl)
              n260 = Add Array Elements(numeric array=w410) -> (sum=w398:dbl)
              n261 = Subtract(x=w399, y=w398) -> (x-y=w397:dbl)
              n262 = Square Root(x=w398) -> (sqrt(x)=w406:dbl)
              n263 = Multiply(x=w405, y=-2.0) -> (x*y=w396:dbl[])
              n264 = Multiply(x=w407, y=w406) -> (x*y=w394:dbl)
              n265 = Build Array (concatenate)(w396, w397) -> (w395:dbl[])
            }
          }
        }
      }
      "circle coeff" <- w246
      "R" <- w245
    }
    frame #3 {
      n266 = global read "G_ALL.vi" "CARSPEC"() -> (w432:T2)
      n267 = Unbundle By Name(w432) -> ("ratio_steer"=w430:dbl, "C_Wheel base"=w431:dbl)
      n268 = local read "R"() -> (w440:dbl)
      n269 = local read "circle point"() -> (w455:dbl[][])
      n270 = global read "G_ALL.vi" "CARDATA"() -> (w443:T1)
      n271 = Divide(x=w431, y=w440) -> (x/y=w438:dbl)
      n272 = Inverse Tangent(1:w438) -> (0:w436:dbl)
      n273 = Unbundle By Name(w443) -> ("VS_can"=w426:dbl)
      n274 = Index Array(array=w455, index (row) #1=0 ("index (row)"), index (row) #2=2 ("disabled index (col)")) -> (element #1=w454:dbl[], element #2=w453:dbl[])  [unwired: 2 in]
      n275 = Multiply(x=-180.0 ("y"), y=w436) -> (x*y=w435:dbl)
      n276 = Subtract(x=w454, y=w453) -> (x-y=w452:dbl[])
      n277 = Divide(x=w426, y=3.6) -> (x/y=w424:dbl)
      n278 = Absolute Value(x=w424) -> (abs(x)=w423:dbl)
      n279 = Index Array(array=w452, index #1=1 ("index"), index #2=0 ("index")) -> (element #1=w449:dbl, element #2=w448:dbl)
      n280 = Divide(x=w435, y=3.141592653589793) -> (x/y=w433:dbl)
      n281 = Inverse Tangent (2 Input)(1:w448, 2:w449) -> (0:w445:dbl)
      n282 = Multiply(x=w430, y=w433) -> (x*y=w439:dbl)
      n283 = Max & Min(x=w423, y=1.0) -> (max(x,y)=w421:dbl)  [unwired: 1 out]
      n284 = Not A Number/Path/Refnum?(number/path/refnum=w439) -> (NaN/Path/Refnum?=w429:bool)
      n285 = local read "x"() -> (w442:dbl)
      n286 = call "headingoperater.vi"("h1"=w445, "h2"=1.5707963267948966) -> ("h2-h1"=w444:dbl)  [unwired: 8 in, 1 out]
      n287 = Divide(x=w442, y=w421) -> (x/y=w441:dbl)
      n288 = Select(t=0.0, s=w429, f=w439) -> (s? t:f=w427:dbl)
      n289 = Build Array(w427, w444, w441) -> (w419:dbl[])
      "ref" <- w419
      n290 = Multiply(x=w419, y="gain") -> (x*y=w417:dbl[])
      n291 = Multiply(x=w417, y=dbl[] [1.0, -1.0, -1.0]) -> (x*y=w415:dbl[])
      n292 = Add Array Elements(numeric array=w415) -> (sum=w418:dbl)
    }
    frame #4 {
      n293 = disable-structure shown="Enabled" {
        disable-tunnel: w461 -> [w486 _]
        disable-tunnel: w460 -> [w484 _]
        frame Enabled {
          w483 = 99999.0 ("upper limit")
          n294 = call "Convert to Dynamic Data5"("Array"=w486) -> ("Dynamic Data Type"=w487:dynamicdata)  [unwired: 3 in]
          n295 = call "Convert to Dynamic Data6"("Array"=w484) -> ("Dynamic Data Type"=w485:dynamicdata)  [unwired: 3 in]
          n296 = local read "circle coeff"() -> (w466:dbl[])
          n297 = Merge Signals(w487, w485) -> (→"Waveform Graph":dynamicdata)
          n298 = Negate(x=w483) -> (-x=w482:dbl)
          n299 = Index Array(array=w466, index #1=0 ("index")) -> (element #1=w464:dbl, element #2=w463:dbl)  [unwired: 1 in]
          n300 = local read "R"() -> (w462:dbl)
          n301 = local read "map_track 2"() -> (w481:dbl[][])
          n302 = local read "circle point"() -> (w478:dbl[][])
          n303 = In Range and Coerce(upper limit=w483, x=w462, lower limit=w482) -> ()  [unwired: 2 out]
          n304 = Polar To Re/Im(2:dbl[] [0.0, 0.017453292519943295, 0.03490658503988659, 0.05235987755982988, 0.06981317007977318, 0.08726646259971647, 0.10471975511965977, 0.12217304763960307, 0.13962634015954636, 0.15707963267948966, 0.17453292519943295, 0.19198621771937624, 0.20943951023931953, 0.22689280275926282, 0.24434609527920614, 0.2617993877991494, 0.2792526803190927, 0.296705972839036, 0.3141592653589793, 0.33161255787892263, 0.3490658503988659, 0.3665191429188092, 0.3839724354387525, 0.40142572795869574, 0.41887902047863906, 0.4363323129985824, 0.45378560551852565, 0.47123889803846897, 0.4886921905584123, 0.5061454830783556, 0.5235987755982988, 0.5410520681182421, 0.5585053606381855, 0.5759586531581287, 0.593411945678072, 0.6108652381980153, 0.6283185307179586, 0.6457718232379019, 0.6632251157578453, 0.6806784082777886, 0.6981317007977318, 0.7155849933176751, 0.7330382858376184, 0.7504915783575618, 0.767944870877505, 0.7853981633974483, 0.8028514559173915, 0.8203047484373349, 0.8377580409572781, 0.8552113334772213, 0.8726646259971648, 0.890117918517108, 0.9075712110370513, 0.9250245035569946, 0.9424777960769379, 0.9599310885968813, 0.9773843811168246, 0.9948376736367678, 1.0122909661567112, 1.0297442586766543, 1.0471975511965976, 1.064650843716541, 1.0821041362364843, 1.0995574287564276, 1.117010721276371, 1.1344640137963142, 1.1519173063162573, 1.1693705988362009, 1.186823891356144, 1.2042771838760875, 1.2217304763960306, 1.239183768915974, 1.2566370614359172, 1.2740903539558606, 1.2915436464758039, 1.3089969389957472, 1.3264502315156905, 1.3439035240356336, 1.3613568165555772, 1.3788101090755203, 1.3962634015954636, 1.413716694115407, 1.4311699866353502, 1.4486232791552935, 1.4660765716752369, 1.48352986419518, 1.5009831567151235, 1.5184364492350666, 1.53588974175501, 1.5533430342749532, 1.5707963267948966, 1.5882496193148399, 1.605702911834783, 1.6231562043547265, 1.6406094968746698, 1.6580627893946132, 1.6755160819145563, 1.6929693744344996, 1.7104226669544427, 1.7278759594743864, 1.7453292519943295, 1.7627825445142729, 1.780235837034216, 1.7976891295541593, 1.8151424220741026, 1.8325957145940461, 1.8500490071139892, 1.8675022996339325, 1.8849555921538759, 1.902408884673819, 1.9198621771937625, 1.9373154697137058, 1.9547687622336491, 1.9722220547535922, 1.9896753472735356, 2.007128639793479, 2.0245819323134224, 2.0420352248333655, 2.0594885173533086, 2.076941809873252, 2.0943951023931953, 2.111848394913139, 2.129301687433082, 2.1467549799530254, 2.1642082724729685, 2.1816615649929116, 2.199114857512855, 2.2165681500327987, 2.234021442552742, 2.251474735072685, 2.2689280275926285, 2.2863813201125716, 2.3038346126325147, 2.321287905152458, 2.3387411976724017, 2.356194490192345, 2.373647782712288, 2.3911010752322315, 2.408554367752175, 2.426007660272118, 2.443460952792061, 2.4609142453120048, 2.478367537831948, 2.495820830351891, 2.5132741228718345, 2.530727415391778, 2.548180707911721, 2.5656340004316642, 2.5830872929516078, 2.600540585471551, 2.6179938779914944, 2.6354471705114375, 2.652900463031381, 2.670353755551324, 2.6878070480712672, 2.705260340591211, 2.7227136331111543, 2.7401669256310974, 2.7576202181510405, 2.7750735106709836, 2.792526803190927, 2.8099800957108707, 2.827433388230814, 2.844886680750757, 2.8623399732707004, 2.8797932657906435, 2.897246558310587, 2.91469985083053, 2.9321531433504737, 2.949606435870417, 2.96705972839036, 2.9845130209103035, 3.001966313430247, 3.01941960595019, 3.036872898470133, 3.0543261909900767, 3.07177948351002, 3.089232776029963, 3.1066860685499065, 3.12413936106985, 3.141592653589793, 3.159045946109736, 3.1764992386296798, 3.193952531149623, 3.211405823669566, 3.2288591161895095, 3.246312408709453, 3.2637657012293966, 3.2812189937493397, 3.2986722862692828, 3.3161255787892263, 3.3335788713091694, 3.3510321638291125, 3.368485456349056, 3.385938748868999, 3.4033920413889422, 3.4208453339088853, 3.4382986264288293, 3.455751918948773, 3.473205211468716, 3.490658503988659, 3.5081117965086026, 3.5255650890285457, 3.543018381548489, 3.560471674068432, 3.5779249665883754, 3.5953782591083185, 3.6128315516282616, 3.630284844148205, 3.647738136668149, 3.6651914291880923, 3.6826447217080354, 3.7000980142279785, 3.717551306747922, 3.735004599267865, 3.752457891787808, 3.7699111843077517, 3.787364476827695, 3.804817769347638, 3.8222710618675815, 3.839724354387525, 3.8571776469074686, 3.8746309394274117, 3.8920842319473548, 3.9095375244672983, 3.9269908169872414, 3.9444441095071845, 3.961897402027128, 3.979350694547071, 3.9968039870670142, 4.014257279586958, 4.031710572106902, 4.049163864626845, 4.066617157146788, 4.084070449666731, 4.101523742186674, 4.118977034706617, 4.136430327226561, 4.153883619746504, 4.171336912266447, 4.1887902047863905, 4.206243497306334, 4.223696789826278, 4.241150082346221, 4.258603374866164, 4.276056667386108, 4.293509959906051, 4.310963252425994, 4.328416544945937, 4.34586983746588, 4.363323129985823, 4.380776422505767, 4.39822971502571, 4.4156830075456535, 4.4331363000655974, 4.4505895925855405, 4.468042885105484, 4.485496177625427, 4.50294947014537, 4.520402762665314, 4.537856055185257, 4.5553093477052, 4.572762640225143, 4.590215932745086, 4.607669225265029, 4.625122517784973, 4.642575810304916, 4.66002910282486, 4.6774823953448035, 4.694935687864747, 4.71238898038469, 4.729842272904633, 4.747295565424576, 4.764748857944519, 4.782202150464463, 4.799655442984406, 4.81710873550435, 4.834562028024293, 4.852015320544236, 4.869468613064179, 4.886921905584122, 4.9043751981040655, 4.9218284906240095, 4.939281783143953, 4.956735075663896, 4.974188368183839, 4.991641660703782, 5.009094953223726, 5.026548245743669, 5.044001538263612, 5.061454830783556, 5.078908123303499, 5.096361415823442, 5.113814708343385, 5.1312680008633285, 5.148721293383272, 5.1661745859032155, 5.183627878423159, 5.201081170943102, 5.218534463463046, 5.235987755982989, 5.253441048502932, 5.270894341022875, 5.288347633542818, 5.305800926062762, 5.323254218582705, 5.340707511102648, 5.358160803622591, 5.3756140961425345, 5.393067388662478, 5.410520681182422, 5.427973973702365, 5.445427266222309, 5.462880558742252, 5.480333851262195, 5.497787143782138, 5.515240436302081, 5.532693728822024, 5.550147021341967, 5.567600313861911, 5.585053606381854, 5.602506898901798, 5.619960191421741, 5.6374134839416845, 5.654866776461628, 5.672320068981571, 5.689773361501514, 5.707226654021458, 5.724679946541401, 5.742133239061344, 5.759586531581287, 5.77703982410123, 5.794493116621174, 5.811946409141117, 5.82939970166106, 5.846852994181004, 5.8643062867009474, 5.8817595792208905, 5.899212871740834, 5.916666164260777, 5.93411945678072, 5.951572749300664, 5.969026041820607, 5.98647933434055, 6.003932626860494, 6.021385919380437, 6.03883921190038, 6.056292504420323, 6.073745796940266, 6.09119908946021, 6.1086523819801535, 6.126105674500097, 6.14355896702004, 6.161012259539983, 6.178465552059926, 6.19591884457987, 6.213372137099813, 6.230825429619757, 6.2482787221397, 6.265732014659643] ("x*y"), 3:w462) -> (0:w474:dbl[], 1:w491:dbl[])
          n305 = Multiply(x=w464, y=-0.5) -> (x*y=w472:dbl)
          n306 = Multiply(x=w463, y=-0.5) -> (x*y=w467:dbl)
          n307 = Add(x=w472, y=w491) -> (x+y=w490:dbl[])
          n308 = Add(x=w474, y=w467) -> (x+y=w469:dbl[])
          n309 = Index Array(array=w481, index (col) #1=0 ("disabled index (col)"), index (col) #2=1 ("disabled index (col)")) -> (element #1=w471:dbl[], element #2=w489:dbl[])  [unwired: 2 in]
          n310 = Index Array(array=w478, index (col) #1=0 ("disabled index (col)"), index (col) #2=1 ("disabled index (col)")) -> (element #1=w470:dbl[], element #2=w475:dbl[])  [unwired: 2 in]
          n311 = call "Convert to Dynamic Data"("Array"=w471) -> ("Dynamic Data Type"=w498:dynamicdata)  [unwired: 3 in]
          n312 = call "Convert to Dynamic Data2"("Array"=w489) -> ("Dynamic Data Type"=w497:dynamicdata)  [unwired: 3 in]
          n313 = call "Convert to Dynamic Data3"("Array"=w490) -> ("Dynamic Data Type"=w495:dynamicdata)  [unwired: 3 in]
          n314 = call "Convert to Dynamic Data4"("Array"=w469) -> ("Dynamic Data Type"=w493:dynamicdata)  [unwired: 3 in]
          n315 = call "Convert to Dynamic Data8"("Array"=w470) -> ("Dynamic Data Type"=w476:dynamicdata)  [unwired: 3 in]
          n316 = call "Convert to Dynamic Data7"("Array"=w475) -> ("Dynamic Data Type"=w477:dynamicdata)  [unwired: 3 in]
          n317 = Merge Signals(w498, w495, w476) -> (w496:dynamicdata)
          n318 = Merge Signals(w497, w493, w477) -> (w494:dynamicdata)
          n319 = call "Build XY Graph"("Y Input"=w494, "X Input"=w496) -> ("XY Graph"=→"XY Graph":cluster{"X":dbl[], "Y":dbl[]}[])  [unwired: 8 in, 1 out]
        }
        frame Disabled {
        }
      }
      "handle" <- w459
    }
  }
